vi "Get Framework Configuration.vi"(8 "error in (no error)":errorcluster, 11 "Item Ref in":T17 format="%.0x") -> (0 "error out":errorcluster, 2 "framework configuration":T1, 3 "Item Ref out":T17 format="%.0x")   [LabVIEW 2020, in "DSF Shared.lvlib"]
uses:
  DSF Shared.lvlib
  <vilib>/NI VeriStand/Custom Device API/Custom Device Item Ref.ctl
  Includes/DSF Core.lvlibp/Typedefs/DSF Engine Framework Configuration.ctl
  Includes/DSF Core.lvlibp/Typedefs/DSF Engine Plugin Configuration.ctl
  Includes/DSF Core.lvlibp/Typedefs/Core Plugin Configuration.ctl
  Includes/DSF Core.lvlibp/Typedefs/DSF Timing Info.ctl
  Includes/DSF Core.lvlibp/Typedefs/DSF Settings Info.ctl
  Includes/DSF Core.lvlibp/Typedefs/DSF Engine Plugin Thread Configuration.ctl
  Includes/DSF Core.lvlibp/Typedefs/Core Thread Configuration.ctl
  Includes/DSF Core.lvlibp/Typedefs/DSF Engine Transfer Group Configuration.ctl
  Includes/DSF Core.lvlibp/Typedefs/Core Group Configuration.ctl
  Includes/DSF Core.lvlibp/Typedefs/DSF Direction.ctl
  Includes/DSF Core.lvlibp/Typedefs/DSF Timeout Behavior.ctl
  Includes/DSF Core.lvlibp/Typedefs/DSF Engine Transfer Configuration.ctl
  Includes/DSF Core.lvlibp/Typedefs/Core Transfer Configuration.ctl
  Includes/DSF Core.lvlibp/Typedefs/DSF Engine Channel Configuration.ctl
  Includes/DSF Core.lvlibp/Typedefs/Core Channel Configuration.ctl
  Includes/DSF Core.lvlibp/Typedefs/DSF Data Type.ctl
  Data Channel Page GUID.vi
  Includes/DSF Core.lvlibp
  Includes/DSF Core.lvlibp/Classes/Configuration/Core/Channel/Channel Configuration.lvclass
  Includes/DSF Core.lvlibp/Classes/Configuration/Core/Transfer/Transfer Configuration.lvclass
  Includes/DSF Core.lvlibp/Classes/Configuration/Core/Group/Group Configuration.lvclass
  Includes/DSF Core.lvlibp/Classes/Configuration/Core/Thread/Thread Configuration.lvclass
  Includes/DSF Core.lvlibp/Classes/Configuration/Core/Plugin/Plugin Configuration.lvclass
  <vilib>/NI VeriStand/Custom Device API/Custom Device API.lvlib
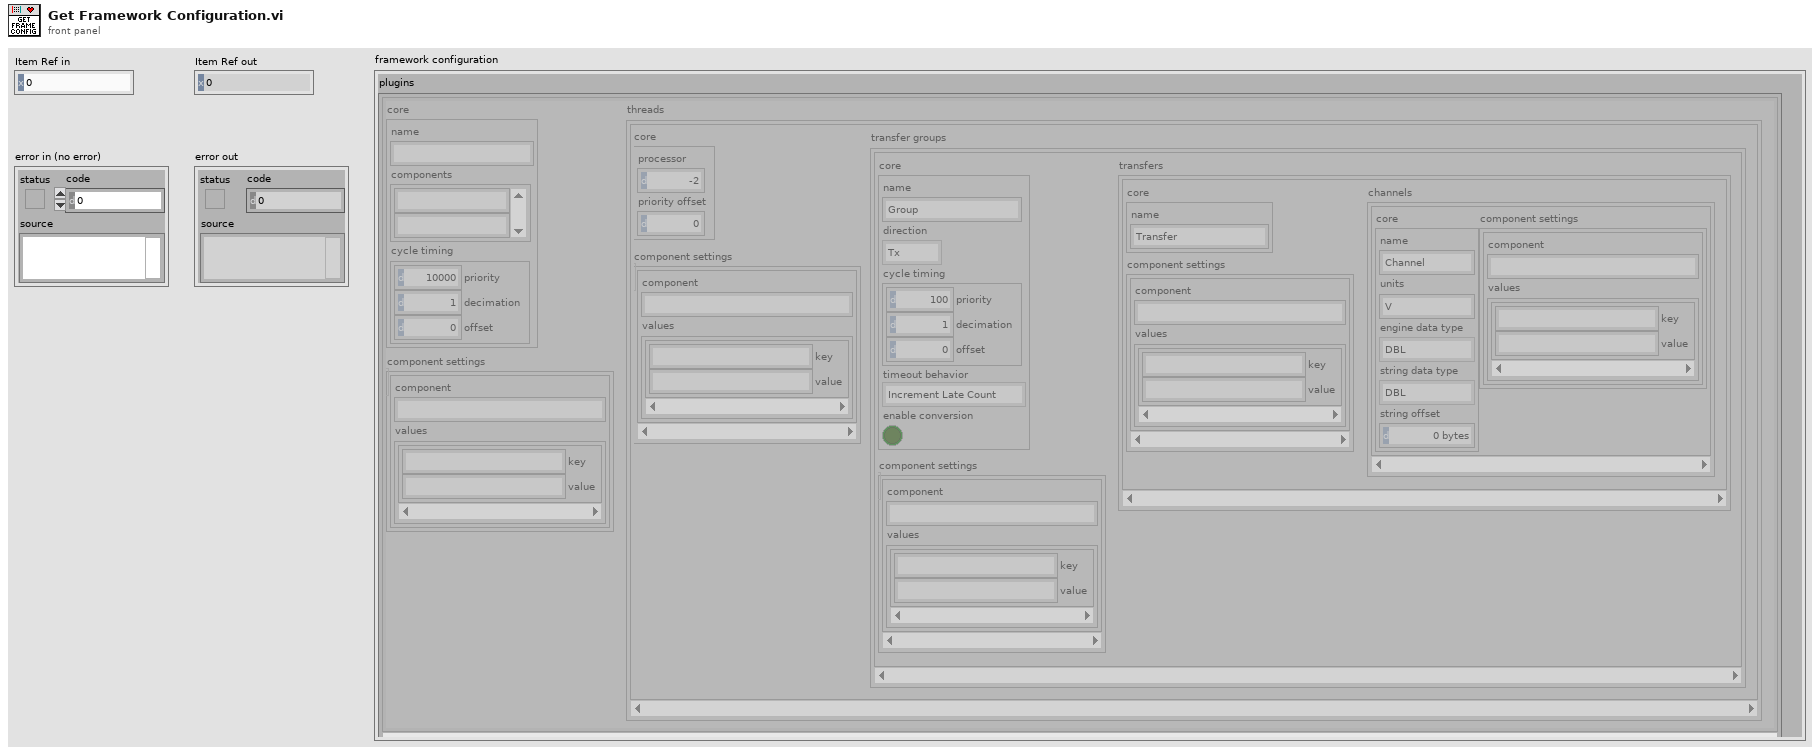
[diagram p1: front panel]
types:
  T1 = typedef "DSF Core.lvlibp/DSF Engine Framework Configuration.ctl" = cluster{"plugins":T2[]}
  T2 = typedef "DSF Core.lvlibp/DSF Engine Plugin Configuration.ctl" = cluster{"core":T3, "component settings":T5[], "threads":T6[]}
  T3 = typedef "DSF Core.lvlibp/Plugin Configuration.lvclass/Core Plugin Configuration.ctl" = cluster{"name":string, "components":string[], "cycle timing":T4}
  T4 = typedef "DSF Core.lvlibp/DSF Timing Info.ctl" = cluster{"priority":u64, "decimation":u64, "offset":u64}
  T5 = typedef "DSF Core.lvlibp/DSF Settings Info.ctl" = cluster{"component":string, "values":cluster{"key":string, "value":string}[]}
  T6 = typedef "DSF Core.lvlibp/DSF Engine Plugin Thread Configuration.ctl" = cluster{"core":T7, "component settings":T5[], "transfer groups":T8[]}
  T7 = typedef "DSF Core.lvlibp/Thread Configuration.lvclass/Core Thread Configuration.ctl" = cluster{"processor":i32, "priority offset":i16}
  T8 = typedef "DSF Core.lvlibp/DSF Engine Transfer Group Configuration.ctl" = cluster{"core":T9, "component settings":T5[], "transfers":T12[]}
  T9 = typedef "DSF Core.lvlibp/Group Configuration.lvclass/Core Group Configuration.ctl" = cluster{"name":string, "direction":T10, "cycle timing":T4, "timeout behavior":T11, "enable conversion":bool}
  T10 = typedef "DSF Core.lvlibp/DSF Direction.ctl" = enum8{"Tx", "Rx"}
  T11 = typedef "DSF Core.lvlibp/DSF Timeout Behavior.ctl" = enum8{"Increment Late Count", "Throw Error"}
  T12 = typedef "DSF Core.lvlibp/DSF Engine Transfer Configuration.ctl" = cluster{"core":T13, "component settings":T5[], "channels":T14[]}
  T13 = typedef "DSF Core.lvlibp/Transfer Configuration.lvclass/Core Transfer Configuration.ctl" = cluster{"name":string}
  T14 = typedef "DSF Core.lvlibp/DSF Engine Channel Configuration.ctl" = cluster{"core":T15, "component settings":T5[]}
  T15 = typedef "DSF Core.lvlibp/Channel Configuration.lvclass/Core Channel Configuration.ctl" = cluster{"name":string, "units":string, "engine data type":T16, "string data type":T16, "string offset":u64}
  T16 = typedef "DSF Core.lvlibp/DSF Data Type.ctl" = enum8{"Bool", "SGL", "DBL", "I8", "I16", "I32", "I64", "U8", "U16", "U32", "U64"}
  T17 = typedef "Custom Device API.lvlib/Custom Device Item Ref.ctl" = u64
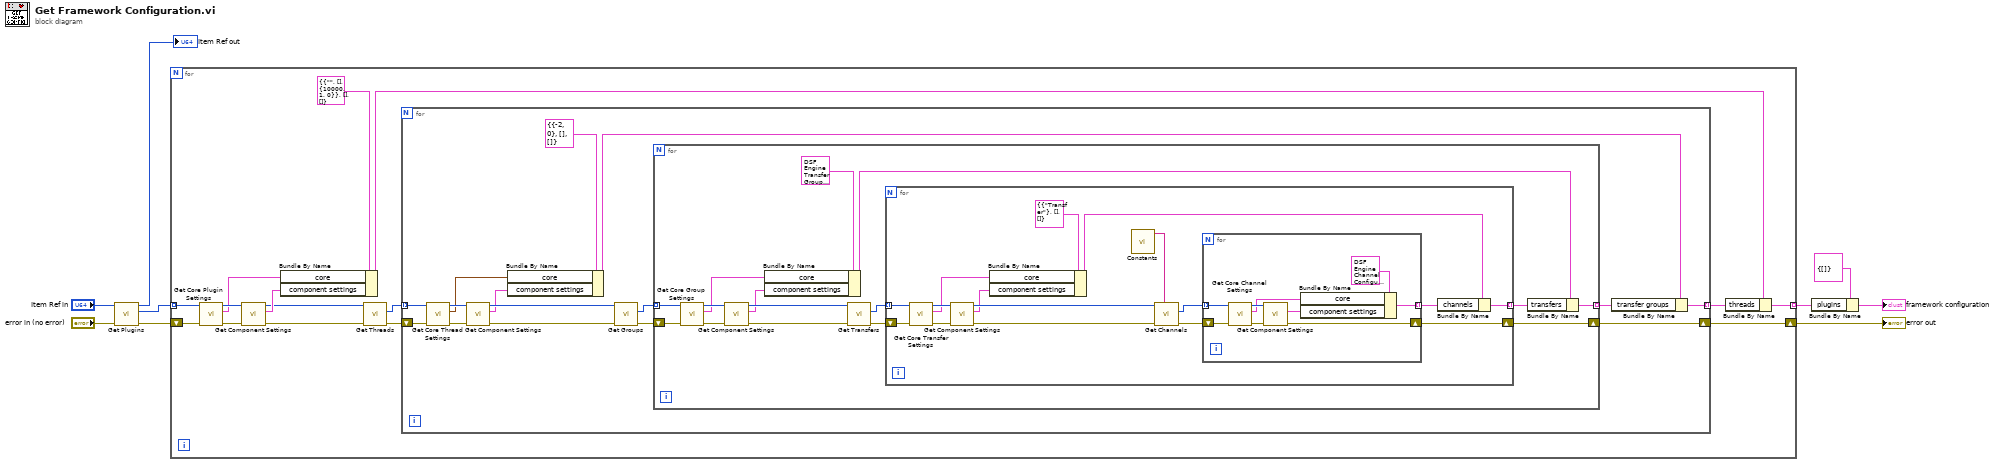
[diagram p0: block diagram]
diagram:
  n1 = call "Get Plugins.vi"("error in (no error)"="error in (no error)", "Item Ref in"="Item Ref in") -> ("error out"=w9:errorcluster, "Plugin refs"=w8:T17[], "Item Ref out"=→"Item Ref out":T17)  [unwired: 7 in]
  n2 = for {
    tunnel: w8 -> [w18] mode=indexing
    shift-right: [w24] -> w2
    shift-left: w9 -> [w19]
    tunnel: [w20] -> w3 mode=indexing
    n3 = call "Get Core Plugin Settings.vi"("error in (no error)"=w19, "Item Ref in"=w18) -> ("error out"=w17:errorcluster, "plugin configuration"=w14:T3, "Item Ref out"=w15:T17)  [unwired: 7 in]
    n4 = call "Get Component Settings.vi"("error in (no error)"=w17, "Item Ref in"=w15) -> ("error out"=w16:errorcluster, "component settings"=w13:T5[], "Item Ref out"=w12:T17)  [unwired: 7 in]
    n5 = Bundle By Name(cluster=T2 {"core"={"name"="", "components"=[], "cycle timing"={"priority"=10000, "decimation"=1, "offset"=0}}, "component settings"=[], "threads"=[]} ("Plugin Configuration"), "core"=w14, "component settings"=w13) -> (w10:T2)
    n6 = call "Get Threads.vi"("error in (no error)"=w16, "Item Ref in"=w12) -> ("error out"=w23:errorcluster, "Plugin refs"=w22:T17[])  [unwired: 7 in, 1 out]
    n7 = for {
      tunnel: w22 -> [w31] mode=indexing
      shift-right: [w35] -> w24
      shift-left: w23 -> [w32]
      tunnel: [w36] -> w21 mode=indexing
      n8 = call "Get Core Thread Settings.vi"("error in (no error)"=w32, "Item Ref in"=w31) -> ("error out"=w30:errorcluster, "thread configuration"=w28:T7, "Item Ref out"=w29:T17)  [unwired: 7 in]
      n9 = call "Get Component Settings.vi"("error in (no error)"=w30, "Item Ref in"=w29) -> ("error out"=w27:errorcluster, "component settings"=w25:T5[], "Item Ref out"=w26:T17)  [unwired: 7 in]
      n10 = Bundle By Name(cluster=T6 {"core"={"processor"=-2, "priority offset"=0}, "component settings"=[], "transfer groups"=[]} ("Plugin Thread Configuration"), "core"=w28, "component settings"=w25) -> (w33:T6)
      n11 = call "Get Groups.vi"("error in (no error)"=w27, "Plugin Ref in"=w26) -> ("error out"=w39:errorcluster, "Group refs"=w38:T17[])  [unwired: 7 in, 1 out]
      n12 = for {
        tunnel: w38 -> [w46] mode=indexing
        shift-right: [w51] -> w35
        shift-left: w39 -> [w47]
        tunnel: [w50] -> w37 mode=indexing
        n13 = call "Get Core Group Settings.vi"("error in (no error)"=w47, "Item Ref in"=w46) -> ("error out"=w45:errorcluster, "group configuration"=w40:T9, "Item Ref out"=w44:T17)  [unwired: 7 in]
        n14 = call "Get Component Settings.vi"("error in (no error)"=w45, "Item Ref in"=w44) -> ("error out"=w43:errorcluster, "component settings"=w41:T5[], "Item Ref out"=w42:T17)  [unwired: 7 in]
        n15 = Bundle By Name(cluster=T8 {"core"={"name"="Group", "direction"=enum."Tx", "cycle timing"={"priority"=100, "decimation"=1, "offset"=0}, "timeout behavior"=enum."Increment Late Count", "enable conversion"=FALSE}, "component settings"=[], "transfers"=[]} ("Transfer Group Configuration"), "core"=w40, "component settings"=w41) -> (w48:T8)
        n16 = call "Get Transfers.vi"("error in (no error)"=w43, "Group Ref in"=w42) -> ("error out"=w54:errorcluster, "Transfer refs"=w53:T17[])  [unwired: 7 in, 1 out]
        n17 = for {
          tunnel: w53 -> [w64] mode=indexing
          shift-right: [w56] -> w51
          shift-left: w54 -> [w66]
          tunnel: [w55] -> w52 mode=indexing
          n18 = call "Get Core Transfer Settings.vi"("error in (no error)"=w66, "Item Ref in"=w64) -> ("error out"=w65:errorcluster, "transfer configuration"=w57:T13, "Item Ref out"=w63:T17)  [unwired: 7 in]
          n19 = call "Get Component Settings.vi"("error in (no error)"=w65, "Item Ref in"=w63) -> ("error out"=w59:errorcluster, "component settings"=w58:T5[], "Item Ref out"=w60:T17)  [unwired: 7 in]
          n20 = Bundle By Name(cluster=T12 {"core"={"name"="Transfer"}, "component settings"=[], "channels"=[]} ("Transfer Configuration"), "core"=w57, "component settings"=w58) -> (w61:T12)
          n21 = call-poly "Constants.vi"() -> ("Status GUID"=w70:string)  [unwired: 11 in]
          n22 = call "Get Channels.vi"("GUID (Default Channel)"=w70, "error in (no error)"=w59, "Item Ref in"=w60) -> ("error out"=w69:errorcluster, "Channels refs"=w68:T17[])  [unwired: 6 in, 1 out]
          n23 = for {
            shift-right: [w75] -> w56
            shift-left: w69 -> [w79]
            tunnel: w68 -> [w78] mode=indexing
            tunnel: [w71] -> w62 mode=indexing
            n24 = call "Get Core Channel Settings.vi"("error in (no error)"=w79, "Item Ref in"=w78) -> ("error out"=w77:errorcluster, "channel configuration"=w72:T15, "Item Ref out"=w76:T17)  [unwired: 7 in]
            n25 = call "Get Component Settings.vi"("error in (no error)"=w77, "Item Ref in"=w76) -> ("error out"=w75:errorcluster, "component settings"=w73:T5[])  [unwired: 7 in, 1 out]
            n26 = Bundle By Name(cluster=T14 {"core"={"name"="Channel", "units"="V", "engine data type"=enum."DBL", "string data type"=enum."DBL", "string offset"=0}, "component settings"=[]} ("channel configuration"), "core"=w72, "component settings"=w73) -> (w71:T14)
          }
          n27 = Bundle By Name(cluster=w61, "channels"=w62) -> (w55:T12)
        }
        n28 = Bundle By Name(cluster=w48, "transfers"=w52) -> (w50:T8)
      }
      n29 = Bundle By Name(cluster=w33, "transfer groups"=w37) -> (w36:T6)
    }
    n30 = Bundle By Name(cluster=w10, "threads"=w21) -> (w20:T2)
  }
  "error out" <- w2
  n31 = Bundle By Name(cluster=T1 {"plugins"=[]} ("framework configuration"), "plugins"=w3) -> (→"framework configuration":T1)
